vi "Constrained IRF Amplitude Array.vi"(8 "Error In":errorcluster, 9 "Independent Last Amplitude":bool, 10 "Time Constant Array":dbl[](array[numeric]), 11 "Amplitude Array":dbl[](array[numeric])) -> (0 "Error Out":errorcluster, 3 "Amplitude Array":dbl[](array[numeric]))   [LabVIEW 2021, in "Fits.lvlib"]
uses:
  Fits.lvlib
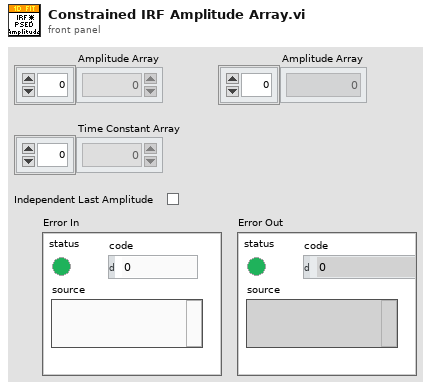
[diagram p1: front panel]
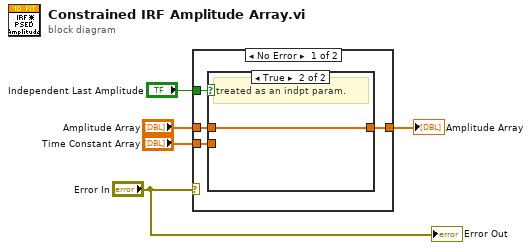
[diagram p0: block diagram]
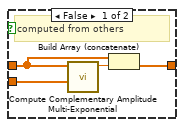
[diagram p2: hidden frame]
diagram:
  n1 = case shown="No Error" "Error In" {
    tunnel: "Time Constant Array" -> [w9 _]
    tunnel: "Amplitude Array" -> [w8 w15]
    tunnel: [w7 w15] -> w3
    tunnel: "Independent Last Amplitude" -> [w6 _]
    frame No Error {
      n2 = case shown="True" w6 {
        tunnel: w9 -> [w13 _]
        tunnel: w8 -> [w12 w14]
        tunnel: [w11 w14] -> w7
        frame False {
          # "computed from others"
          n3 = call "Compute Complementary Amplitude Multi-Exponential.vi"("Time Constant Array"=w13, "Amplitude Array"=w12) -> ("Complementary Amplitude"=w10:dbl)  [unwired: 8 in, 1 out]
          n4 = Build Array (concatenate)(w12, w10) -> (w11:dbl[])
        }
        frame True {
          # "treated as an indpt param."
        }
      }
    }
    frame Error {
    }
  }
  "Amplitude Array" <- w3
  "Error Out" <- "Error In"
